vi "Self Queue Alias.vi"(11 "qqqqq in":refnum<class "qqqqq.lvclass">) -> (2 "Self Queue Alias":string)   [LabVIEW 2021, in "jettl Tools.lvlib" / "qqqqq.lvlib" / "qqqqq.lvclass"]
uses:
  qqqqq.lvclass
  qqqqq.lvclass/qqqqq.ctl
  jettl/Queue/Queue.lvclass
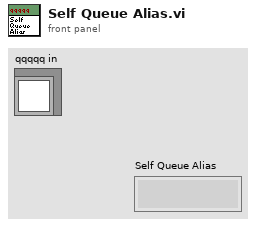
[diagram p1: front panel]
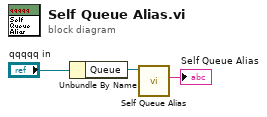
[diagram p0: block diagram]
diagram:
  n1 = Unbundle By Name("qqqqq in") -> ("Queue"=w2:refnum<class "Queue.lvclass">)
  n2 = call-dynamic "Self Queue Alias.vi"("Queue in"=w2) -> ("Self Queue Alias"=→"Self Queue Alias":string)  [unwired: 10 in]
